vi "deinitialize.vi"(0 "HGF_ImaqFg":refnum<class "HGF_ImaqUsb.lvclass">, 5 "error in (no error)":errorcluster) -> (19 "error out":errorcluster)   [LabVIEW 2009, in "HGF_ImaqUsb.lvclass"]
doc: "This is a dynamic dispatch VI. It can be overwritten by childclasses to release allocated recources."
uses:
  HGF_ImaqUsb.lvclass
  HGF_IMAQDevice/HGF_IMAQDevice.lvclass
  HGF_ImaqUsb.lvclass/HGF_ImaqUsb.ctl
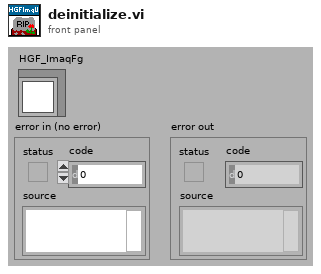
[diagram p1: front panel]
types:
  T1 = typedef "IMAQ USB.ctl" = refnum<k1>
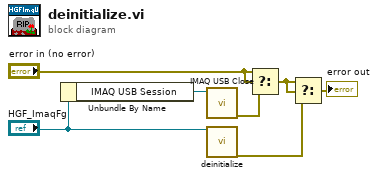
[diagram p0: block diagram]
diagram:
  n1 = Unbundle By Name("HGF_ImaqFg") -> ("IMAQ USB Session"=w1:T1)
  n2 = call <vilib>:"IMAQ USB Close.vi"("IMAQ USB Session In"=w1) -> ("error out"=w2:errorcluster)  [unwired: 1 in, 9 out]
  n3 = call-parent "deinitialize.vi"("HGF_IMAQDevice"="HGF_ImaqFg") -> ("error out"=w4:errorcluster)  [unwired: 1 in, 17 out]
  n4 = Select(t="error in (no error)", s="error in (no error)", f=w2) -> (s? t:f=w5:errorcluster)
  n5 = Select(t=w5, s=w5, f=w4) -> (s? t:f=→"error out":errorcluster)
